vi "Demo_DownloadSTLFile.vi"   [LabVIEW 2019]
uses:
  <userlib>/Onshape/_SubVI/z did wid and eid.vi
types:
  T1 = typedef "Cluster.ctl" = cluster{"Date":string, "On-Nonce":string, "eid":string, "wid":string, "did":string, "name":string, "method":string, "Accept":string, "User-Agent":string, "Content-Type":string, "stack":string, "headers":string[], "payload":string, "addition":string, "path":string, "Authorization":string, "secret_key":string, "access_key":string}
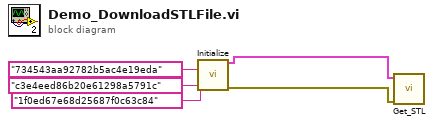
[diagram p0: block diagram]
diagram:
  n1 = call-poly <userlib>:"Initialize.vi"("did"="734543aa92782b5ac4e19eda", "wid"="c3e4eed86b20e61298a5791c", "eid"="1f0ed67e68d25687f0c63c84") -> ("Device Out"=w5:T1, "error out"=w4:errorcluster)  [unwired: 11 in]
  n2 = call <userlib>:"Get_STL.vi"("error in"=w4, "Device In"=w5) -> ()  [unwired: 6 in, 4 out]
